vi "Home_u_0.vi"() -> ()   [LabVIEW 2011]
uses:
  Globals/Global Recipe.vi
  Globals/Global VI.vi
panel:
  in  "Stop Button":bool
  in  "Pause Button":bool
  in  "Play Button":bool
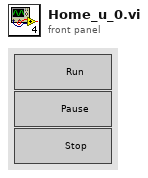
[diagram p1: front panel]
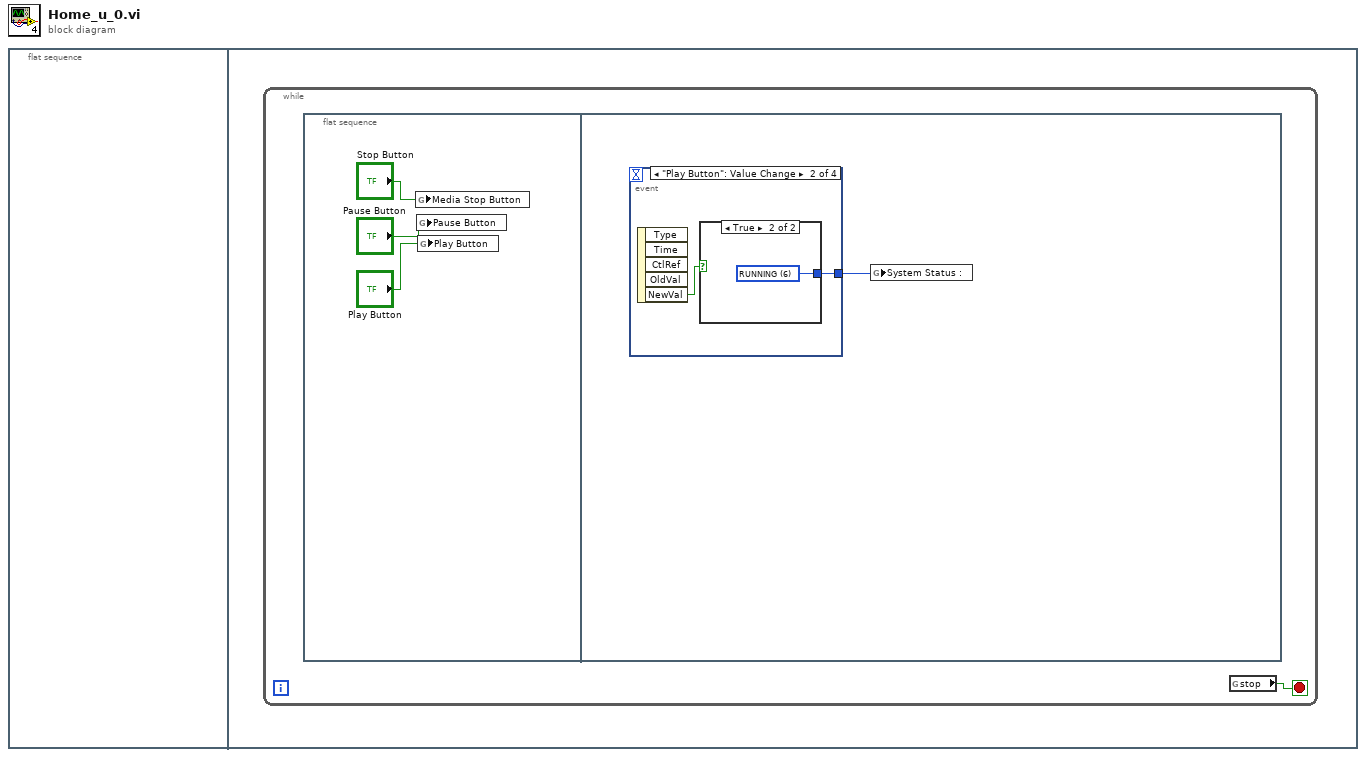
[diagram p0: block diagram]
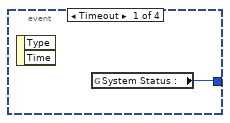
[diagram p2: hidden frame]
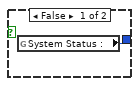
[diagram p3: hidden frame]
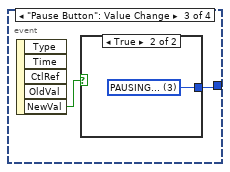
[diagram p4: hidden frame]
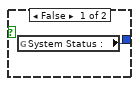
[diagram p5: hidden frame]
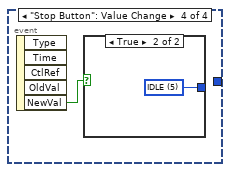
[diagram p6: hidden frame]
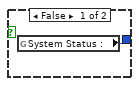
[diagram p7: hidden frame]
diagram:
  n1 = flat-sequence {
    frame #0 {
    }
    frame #1 {
      n2 = while {
        stop <- w1 stop-if-true
        n3 = flat-sequence {
          frame #0 {
            n4 = global write "Global Recipe.vi" "Media Stop Button"("Stop Button") -> ()
            n5 = global write "Global Recipe.vi" "Pause Button"("Pause Button") -> ()
            n6 = global write "Global Recipe.vi" "Play Button"("Play Button") -> ()
          }
          frame #1 {
            n7 = event shown="[1] \"Play Button\": Value Change" {
              selector: _ -> [_ _ _ _]
              dyn-events: _ -> [_ _ _ _]
              timeout: _ -> [_ _ _ _]
              tunnel: [w6 w7 w11 _] -> w5
              event Timeout {
                n8 = event-data() -> ()  [unwired: 1 in, 2 out]
                n9 = global read "Global Recipe.vi" "System Status :"() -> (w6:u16)
              }
              event "Play Button": Value Change {
                n10 = event-data() -> ("NewVal"=w8:bool)  [unwired: 1 in, 4 out]
                n11 = case shown="True" w8 {
                  tunnel: [w9 w10] -> w7
                  frame False {
                    n12 = global read "Global Recipe.vi" "System Status :"() -> (w9:u16)
                  }
                  frame True {
                    w10 = u16 6 items=["NOT READY", "E-STOPPED", "FAULTED", "PAUSING...", "PAUSED", "IDLE", "RUNNING", "UNCALIBRATED", "CALIBRATING...", "POWER OFF", "POWERING ON...", "MANUAL MODE", "CONNECTING..."] ("System Status :")
                  }
                }
              }
              event "Pause Button": Value Change {
                n13 = event-data() -> ("NewVal"=w12:bool)  [unwired: 1 in, 4 out]
                n14 = case shown="True" w12 {
                  tunnel: [w13 w14] -> w11
                  frame False {
                    n15 = global read "Global Recipe.vi" "System Status :"() -> (w13:u16)
                  }
                  frame True {
                    w14 = u16 3 items=["NOT READY", "E-STOPPED", "FAULTED", "PAUSING...", "PAUSED", "IDLE", "RUNNING", "UNCALIBRATED", "CALIBRATING...", "POWER OFF", "POWERING ON...", "MANUAL MODE", "CONNECTING..."] ("System Status :")
                  }
                }
              }
              event "Stop Button": Value Change {
                n16 = event-data() -> ("NewVal"=w15:bool)  [unwired: 1 in, 4 out]
                n17 = case shown="True" w15 {
                  tunnel: [w16 w17] -> _
                  frame False {
                    n18 = global read "Global Recipe.vi" "System Status :"() -> (w16:u16)
                  }
                  frame True {
                    w17 = u16 5 items=["NOT READY", "E-STOPPED", "FAULTED", "PAUSING...", "PAUSED", "IDLE", "RUNNING", "UNCALIBRATED", "CALIBRATING...", "POWER OFF", "POWERING ON...", "MANUAL MODE", "CONNECTING..."] ("System Status :")
                  }
                }
              }
            }
            n19 = global write "Global Recipe.vi" "System Status :"(w5) -> ()
          }
        }
        n20 = global read "Global VI.vi" "stop"() -> (w1:bool)
      }
    }
  }
